vi "数据输出.vi"() -> ()   [LabVIEW 2018]
panel:
  out "字符串":string
  out "数值":dbl
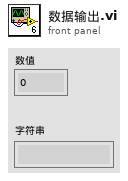
[diagram p1: front panel]
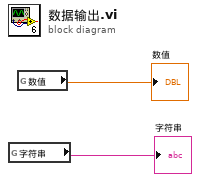
[diagram p0: block diagram]
diagram:
  n1 = global read "全局变量.vi" "字符串"() -> (→"字符串":string)
  n2 = global read "全局变量.vi" "数值"() -> (→"数值":dbl)
